vi "InitFromPPL.vi"(8 "error in (no error)":errorcluster, 10 "qualified name":string, 11 "packed library path":path) -> (0 "error out":errorcluster, 3 "AbstractCalc out":refnum<class "AbstractCalc.lvclass">)   [LabVIEW 2015, in "AbstractCalcLib.lvlib" / "AbstractCalc.lvclass"]
uses:
  AbstractCalc.lvclass
  <vilib>/Utility/error.llb/Error Cluster From Error Code.vi
  <vilib>/ErrorRing/Error Ring.xnode
  <vilib>/Utility/LVLibp/NI_PackedLibraryUtility.lvlib
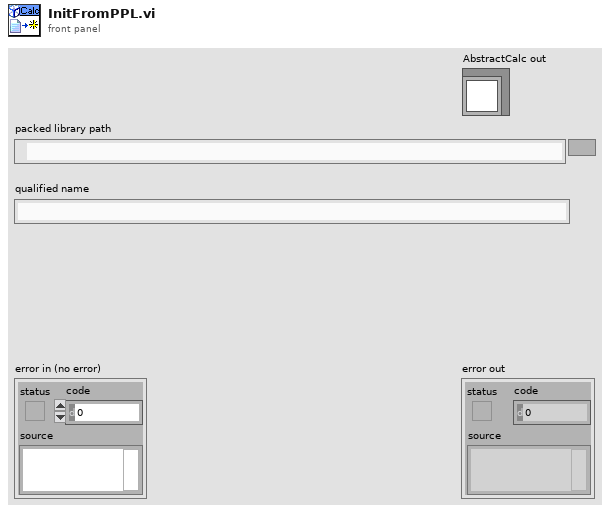
[diagram p1: front panel]
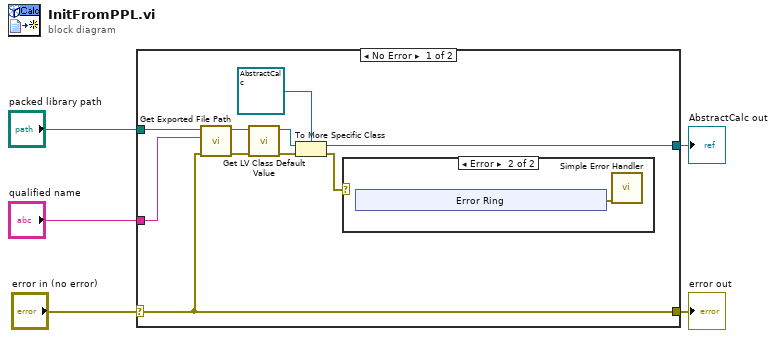
[diagram p0: block diagram]
diagram:
  n1 = case shown="No Error" "error in (no error)" {
    selector: "error in (no error)" -> [w7 w22]
    tunnel: [w7 w22] -> w4
    tunnel: [w9 _] -> w1
    tunnel: "packed library path" -> [w11 _]
    tunnel: "qualified name" -> [w10 _]
    frame No Error {
      n2 = call <vilib>:"Get Exported File Path.vi"("error in (no error)"=w7, "qualified name"=w10, "packed library path"=w11) -> ("error out"=w15:errorcluster, "path"=w14:path)  [unwired: 7 in]
      n3 = call <vilib>:"Get LV Class Default Value.vi"("error in (no error)"=w15, "class path"=w14) -> ("error out"=w13:errorcluster, "object"=w12:refnum<class>)  [unwired: 8 in]
      n4 = To More Specific Class(target class=refnum<class "AbstractCalc.lvclass"> refnum ("AbstractCalc in"), reference=w12, error in=w13) -> (specific class reference=w9:refnum<class "AbstractCalc.lvclass">, error out=w6:errorcluster)
      n5 = case shown="Error" w6 {
        frame No Error {
        }
        frame Error {
          n6 = xnode "Error Ring"() -> ("error out"=w16:errorcluster)
          n7 = call <vilib>:"Simple Error Handler.vi"("error in (no error)"=w16) -> ()  [unwired: 4 in, 5 out]
        }
      }
    }
    frame Error {
    }
  }
  "error out" <- w4
  "AbstractCalc out" <- w1
